vi "WaitOccurence.vi"(11 "occurence":i32) -> (3 "timeout":i32)   [LabVIEW 2011]
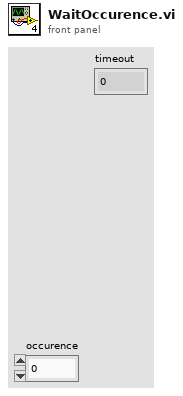
[diagram p1: front panel]
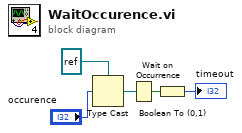
[diagram p0: block diagram]
diagram:
  n1 = Type Cast(type=refnum<k4> refnum ("事件发生"), x="occurence") -> (*(type *) &x=w3:refnum<k4>)
  n2 = Wait on Occurrence(2:w3) -> (0:w2:bool)  [unwired: 2 in]
  n3 = Boolean To (0,1)(Boolean=w2) -> (0, 1=→"timeout":i16)
